vi "UI Refresh Data.vi"(8 "error in (no error)":errorcluster, 11 "GObject View in":refnum<class "GObject View.lvclass">) -> (0 "error out":errorcluster, 3 "GObject View out":refnum<class "GObject View.lvclass">)   [LabVIEW 2013, in "SET Project Editor.lvlib" / "GObject View.lvclass"]
uses:
  GObject View.lvclass
  UI View/UI View.lvclass/UI View.ctl
  GObject View.lvclass/GObject View.ctl
  SET Project Data/Project Data Class/Project Data.lvclass
  SET Project Data/VI Class/VI Data.lvclass
  SET Project Data/Control Classes/GObject/GObject.lvclass/GObject.ctl
  UI View/Read _LangData.vi
  UI View/Read UUID.vi
  SET Project Data/Control Classes/GObject/Read Items.vi
  SET Project Data/Control Classes/GObject/Read UID.vi
  SET Project Data/Control Classes/GObject/Read Label.vi
  SET Project Data/Control Classes/GObject/Read Owning VI.vi
  SET Project Data/Control Classes/GObject/Read ClassName.vi
  SET Project Data/Control Classes/GObject/Read Languages.vi
  SET Project Editor.lvlib
  SET Project Data/Control Classes/GObject/GObject.lvclass
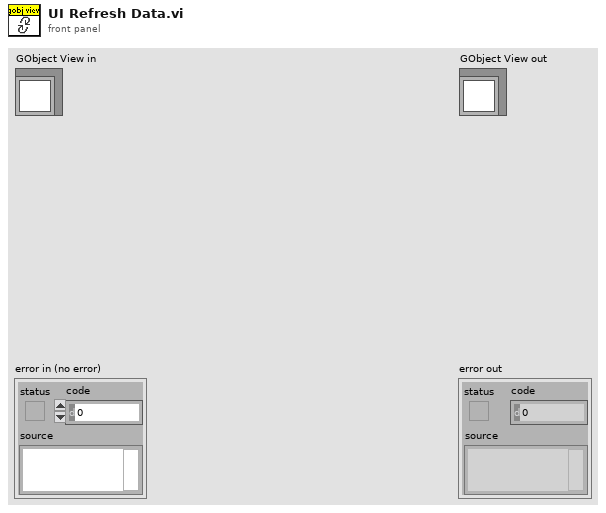
[diagram p1: front panel]
types:
  T1 = typedef "SET Resource File.lvlib/ResFile Lang Entry.ctl" = cluster{"Tag":string, "Name":string, "Code Page":u16}
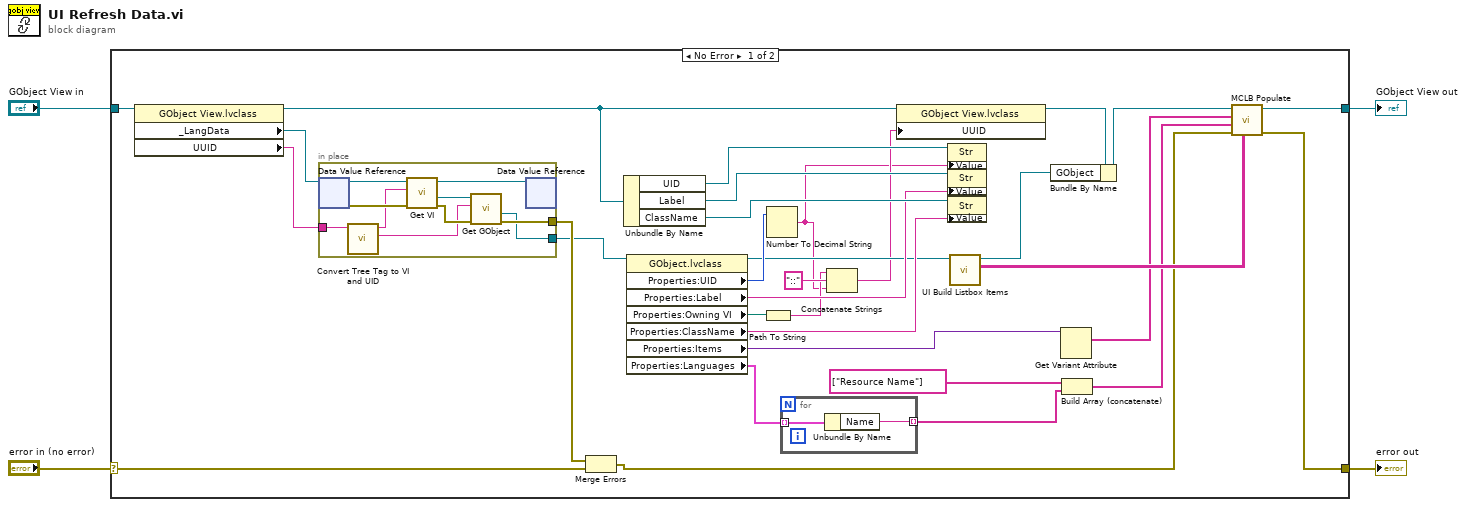
[diagram p0: block diagram]
diagram:
  n1 = case shown="No Error" "error in (no error)" {
    selector: "error in (no error)" -> [w20 w50]
    tunnel: [w17 w50] -> w3
    tunnel: [w16 w49] -> w1
    tunnel: "GObject View in" -> [w36 w49]
    frame No Error {
      n2 = property class="GObject View.lvclass"(reference=w36) -> (reference out=w13:refnum<class "GObject View.lvclass">, "_LangData"=w35:refnum<data-value>, "UUID"=w34:string)  [unwired: 1 in, 1 out]
      n3 = in-place {
        in-place-border: [w44] -> w33
        in-place-border: w34 -> [w42]
        in-place-border: [w39] -> w19
        n4 = in-place-dvr #1(w35) -> (w48:refnum<class "Project Data.lvclass">, w43:errorcluster)
        n5 = call "Convert Tree Tag to VI and UID.vi"("Tree Tag"=w42) -> ("GObject UID"=w40:string, "File Path (Relative)"=w41:string)  [unwired: 7 in, 2 out]
        n6 = call-dynamic "Get VI.vi"("error in (no error)"=w43, "VI Path (Relative)"=w41, "ProjectData in"=w48) -> ("error out"=w45:errorcluster, "VI Data out"=w47:refnum<class "VI Data.lvclass">, "ProjectData out"=w46:refnum<class "Project Data.lvclass">)  [unwired: 5 in, 1 out]
        n7 = call-dynamic "Get GObject.vi"("error in (no error)"=w45, "GObject UID"=w40, "VI Data in"=w47) -> ("error out"=w44:errorcluster, "GObject"=w39:refnum<class "GObject.lvclass">)  [unwired: 5 in, 2 out]
        n8 = in-place-dvr #1(w46) -> ()  [unwired: 2 out]
      }
      n9 = Merge Errors(w33, w20) -> (w18:errorcluster)
      n10 = Unbundle By Name(w13) -> ("UID"=w32:refnum<vi>, "Label"=w31:refnum<vi>, "ClassName"=w30:refnum<vi>)
      n11 = property class="GObject.lvclass"(reference=w19) -> (reference out=w24:refnum<class "GObject.lvclass">, "Properties:UID"=w27:i32, "Properties:Label"=w29:string, "Properties:Owning VI"=w11:path, "Properties:ClassName"=w28:string, "Properties:Items"=w25:variant, "Properties:Languages"=w6:T1[])  [unwired: 1 in, 1 out]
      n12 = Path To String(path=w11) -> (string=w8:string)
      n13 = Number To Decimal String(number=w27) -> (decimal integer string=w7:string)  [unwired: 1 in]
      n14 = for {
        tunnel: w6 -> [w38] mode=indexing
        tunnel: [w37] -> w5 mode=indexing
        n15 = Unbundle By Name(w38) -> ("Name"=w37:string)
      }
      n16 = Concatenate Strings(w8, "::" ("string"), w7) -> (w9:string)
      n17 = property class="GObject View.lvclass"(reference=w13, "UUID"=w9) -> (reference out=w12:refnum<class "GObject View.lvclass">)  [unwired: 1 in, 1 out]
      n18 = property class="Str"(reference=w32, "Value"=w7) -> ()  [unwired: 1 in, 2 out]
      n19 = property class="Str"(reference=w31, "Value"=w29) -> ()  [unwired: 1 in, 2 out]
      n20 = property class="Str"(reference=w30, "Value"=w28) -> ()  [unwired: 1 in, 2 out]
      n21 = call "UI Build Listbox Items.vi"("GObject in"=w24) -> ("GObject Item Strings (UTF-16)"=w23:string[][], "GObject out"=w14:refnum<class "GObject.lvclass">)  [unwired: 8 in, 1 out]
      n22 = Bundle By Name(cluster=w12, "GObject"=w14) -> (w15:refnum<class "GObject View.lvclass">)
      n23 = Get Variant Attribute(Variant=w25) -> (names=w21:string[])  [unwired: 3 in, 3 out]
      n24 = Build Array (concatenate)(string[] ["Resource Name"], w5) -> (w22:string[])
      n25 = call-dynamic "MCLB Populate.vi"("Item Names[][]"=w23, "error in (no error)"=w18, "Column Header Strings[]"=w22, "Row Header Strings[]"=w21, "View in"=w15) -> ("error out"=w17:errorcluster, "View out"=w16:refnum<class "GObject View.lvclass">)  [unwired: 5 in]
    }
    frame Error {
    }
  }
  "error out" <- w3
  "GObject View out" <- w1
